vi "Autonomous Independent.vi"() -> ()   [LabVIEW 2015]
doc: "This VI is called when autonomous begins, and will automatically be terminated when autonomous ends. You can carry out timed or sensor driven robot movement independently without needing to return to the caller."
uses:
  <vilib>/Rock Robotics/SystemInterfaces/i2clib/i2c_bus.ctl
  <vilib>/Rock Robotics/Network Tables/NT Read String.vi
  <vilib>/Rock Robotics/WPI/Utilities/WPI_GetSetVariantRefNum.vi
  navX-MXP-LabVIEW/navX Library v2/navX Library v2.lvlib
panel:
  in  "array":bool[](array[boolean])
  in  "Distance (ft) 2":dbl
  in  "Angle (degrees)":dbl format="%.2f"
  in  "Distance (ft)":dbl
  # "Go this far"
  # "Turn thusly"
  # "Be sure to right-click and choose Data Operations>>Make Current Value default if you want to save the array values with the VI"
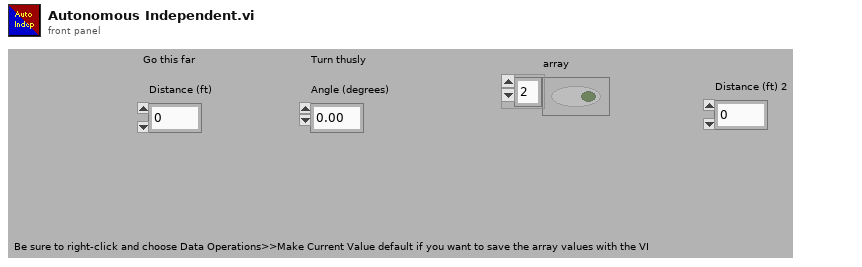
[diagram p1: front panel]
types:
  T1 = typedef "i2c_bus.ctl" = enum16{"I2C On-Board", "I2C MXP", "Invalid"}
  T2 = typedef "navX Library v2.lvlib/Z900_navX_DeviceTypeDef.ctl" = cluster{"Interface":cluster{"Protocol":T3, "Update Rate (4Hz-60Hz)":u8, "navX Open TypeDef":variant}, "Notify Packet":refnum<notifier>, "Loop VI Refnum":refnum<vi>, "Ready to Close Occurrence Refnum":refnum<k4>}
  T3 = typedef "navX Library v2.lvlib/Z900_navX_ProtocolTypeDef.ctl" = enum16{"SERIAL", "I2C", "SPI"}
  T4 = typedef "WPI_RobotDriveDevRef.ctl" = cluster{"DevStatus":errorcluster, "Motors[]":T5[], "Square Inputs":bool, "Max Output":dbl}
  T5 = typedef "WPI_MotorControlDeviceRef.ctl" = cluster{"DeviceStatus":errorcluster, "Type":T6, "PWM":cluster{"PWM Channel":T7, "DeadBand":T8}, "CAN":cluster{"Device Number":u8, "Control Mode":T9, "Semaphore":T10, "Max Vout":dbl, "TalonSRX Control Mode":T11}, "Invert":bool}
  T6 = typedef "WPI_MotorControlType.ctl" = enum16{"PWM", "CAN", "CANTalonSRX"}
  T7 = typedef "FPGA_DIOPWMChannel.ctl" = enum8{"PWM 0", "PWM 1", "PWM 2", "PWM 3", "PWM 4", "PWM 5", "PWM 6", "PWM 7", "PWM 8", "PWM 9", "PWM MXP 0", "PWM MXP 1", "PWM MXP 2", "PWM MXP 3", "PWM MXP 4", "PWM MXP 5", "PWM MXP 6", "PWM MXP 7", "PWM MXP 8", "PWM MXP 9", "Invalid"}
  T8 = typedef "WPI_PWMDeadband.ctl" = cluster{"Name":string, "maxPositivePwm":i32, "minPositivePwm":i32, "centerPwm":i32, "maxNegativePwm":i32, "minNegativePwm":i32, "angularRange":u16}
  T9 = typedef "WPI_CANJaguar_ControlMode.ctl" = enum8{"Percent VBus", "Current", "Speed", "Position", "Voltage"}
  T10 = typedef "Semaphore RefNum" = refnum<k1>
  T11 = typedef "WPI_CANTalonSRX_APIControlMode.ctl" = enum8{"Percent VBus", "Speed", "Position", "Slave", "Unchanged / Invalid", "Voltage Compensation", "Current", "Motion Profile"}
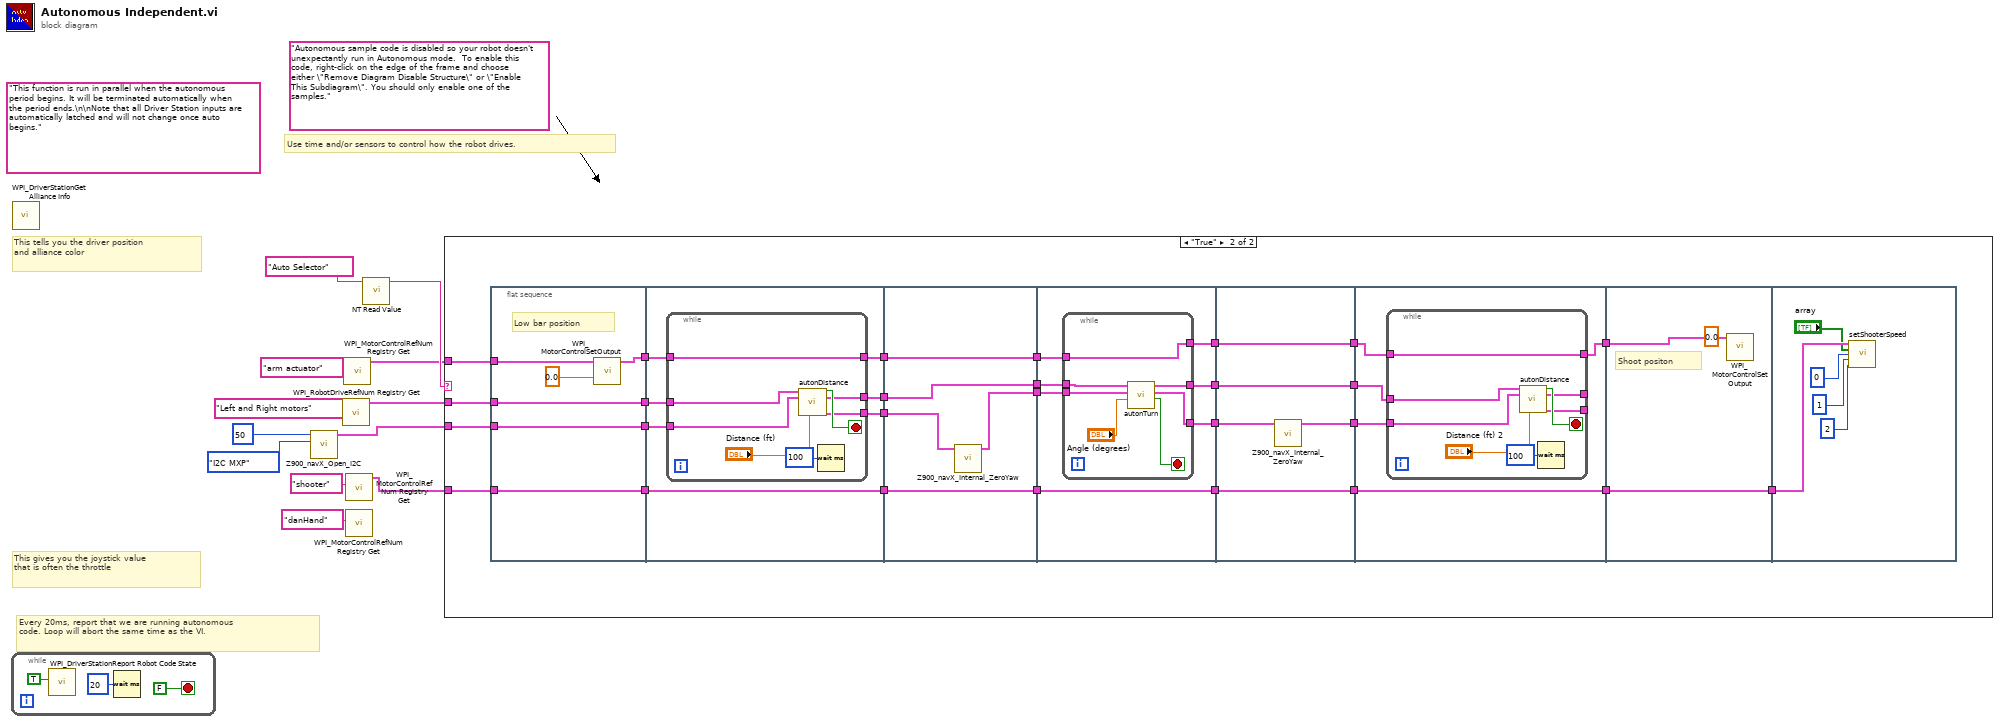
[diagram p0: block diagram]
diagram:
  (unwired) "Autonomous sample code is disabled so your robot doesn't unexpectantly run in Autonomous mode.  To enable this code, right-click on the edge of the frame and choose either \"Remove Diagram Disable Structure\" or \"Enable This Subdiagram\". You should only enable one of the samples."
  (unwired) "This function is run in parallel when the autonomous period begins. It will be terminated automatically when the period ends.\n\nNote that all Driver Station inputs are automatically latched and will not change once auto begins."
  # "Every 20ms, report that we are running autonomous\ncode. Loop will abort the same time as the VI."
  # "This gives you the joystick value\nthat is often the throttle"
  # "Use time and/or sensors to control how the robot drives."
  # "This tells you the driver position\nand alliance color"
  n1 = while {
    stop <- FALSE stop-if-true
    n2 = call <vilib>:"WPI_DriverStationReport Robot Code State.vi"("Autonomous"=TRUE) -> ()  [unwired: 10 in, 1 out]
    n3 = Wait (ms)(milliseconds to wait=u32 20) -> ()  [unwired: 1 out]
  }
  n4 = call <vilib>:"WPI_DriverStationGet Alliance Info.vi"() -> ()  [unwired: 12 out]
  n5 = call "Z900_navX_Open_I2C.vi"("I2C Bus"=i2c_bus."I2C MXP", "Update Rate (4Hz-60Hz)"=u8 50) -> ("navX Device"=w3:T2)  [unwired: 8 in, 1 out]
  n6 = call <vilib>:"WPI_RobotDriveRefNum Registry Get.vi"("refnum name"="Left and Right motors") -> ("RobotDriveDevRef"=w9:T4)  [unwired: 9 in, 1 out]
  n7 = call <vilib>:"WPI_MotorControlRefNum Registry Get.vi"("refnum name"="arm actuator") -> ("MotorControlDevRef"=w7:T5)  [unwired: 9 in, 1 out]
  n8 = call <vilib>:"WPI_MotorControlRefNum Registry Get.vi"("refnum name"="shooter") -> ("MotorControlDevRef"=w4:T5)  [unwired: 9 in, 1 out]
  n9 = call <vilib>:"WPI_MotorControlRefNum Registry Get.vi"("refnum name"="danHand") -> ()  [unwired: 9 in, 2 out]
  n10 = call-poly <vilib>:"NT Read Value.vi"("Name"="Auto Selector") -> ("String"=w11:string)  [unwired: 9 in, 1 out]
  n11 = case shown="\"True\"" w11 {
    tunnel: w9 -> [_ w42]
    tunnel: w3 -> [_ w41]
    tunnel: w7 -> [_ w24]
    tunnel: w4 -> [_ w23]
    frame "False", Default {
    }
    frame "True" {
      n12 = flat-sequence {
        tunnel: w41 -> [w47]
        tunnel: w42 -> [w48]
        tunnel: [w48] -> w27
        tunnel: [w47] -> w26
        tunnel: [w46] -> w25
        tunnel: w24 -> [w45]
        tunnel: w23 -> [w44]
        tunnel: [w44] -> w22
        tunnel: [w53] -> w40
        tunnel: [w52] -> w37
        tunnel: [w51] -> w35
        tunnel: w27 -> [w55]
        tunnel: w26 -> [w54]
        tunnel: w25 -> [w50]
        tunnel: w22 -> [w49]
        tunnel: [w49] -> w21
        tunnel: w40 -> [w65]
        tunnel: [w64] -> w39
        tunnel: [w68] -> w38
        tunnel: w37 -> [w68]
        tunnel: [w67] -> w36
        tunnel: w35 -> [w67]
        tunnel: w21 -> [w66]
        tunnel: [w66] -> w20
        tunnel: w39 -> [w75]
        tunnel: w38 -> [w74]
        tunnel: [w73] -> w33
        tunnel: w36 -> [w72]
        tunnel: [w71] -> w31
        tunnel: [w70] -> w29
        tunnel: w20 -> [w69]
        tunnel: [w69] -> w19
        tunnel: w33 -> [w87]
        tunnel: [w87] -> w32
        tunnel: w31 -> [w86]
        tunnel: [w86] -> w30
        tunnel: w29 -> [w84]
        tunnel: [w83] -> w28
        tunnel: w19 -> [w85]
        tunnel: [w85] -> w18
        tunnel: w32 -> [w92]
        tunnel: [w89] -> w34
        tunnel: w30 -> [w91]
        tunnel: w28 -> [w90]
        tunnel: w18 -> [w88]
        tunnel: [w88] -> w17
        tunnel: w34 -> [w103]
        tunnel: w17 -> [w102]
        tunnel: [w102] -> w16
        tunnel: w16 -> [w108]
        frame #0 {
          # "Low bar position"
          n13 = call <vilib>:"WPI_MotorControlSetOutput.vi"("Output"=0.0, "MotorControlDevRef"=w45) -> ("MotorControlDevRef"=w46:T5)  [unwired: 7 in, 2 out]
        }
        frame #1 {
          n14 = while {
            tunnel: w55 -> [w60]
            tunnel: w54 -> [w59]
            tunnel: [w58] -> w53
            tunnel: [w57] -> w52
            tunnel: [w56] -> w51
            tunnel: w50 -> [w56]
            stop <- w63 stop-if-true
            n15 = call "autonDistance.vi"("RobotDriveDevRef"=w60, "navX Device"=w59, "Numeric"="Distance (ft)") -> ("s? t:f"=w63:bool, "RobotDriveDevRef 2"=w57:T4, "navX Device 2"=w58:T2)  [unwired: 8 in, 2 out]
            n16 = Wait (ms)(milliseconds to wait=u32 100) -> ()  [unwired: 1 out]
          }
        }
        frame #2 {
          n17 = call "Z900_navX_Internal_ZeroYaw.vi"("navX Device"=w65) -> ("navX Device"=w64:T2)  [unwired: 7 in, 3 out]
        }
        frame #3 {
          n18 = while {
            tunnel: w75 -> [w82]
            tunnel: w74 -> [w81]
            tunnel: [w78] -> w73
            tunnel: w72 -> [w78]
            tunnel: [w77] -> w71
            tunnel: [w76] -> w70
            stop <- w79 stop-if-true
            n19 = call "autonTurn.vi"("setpoint"="Angle (degrees)", "navX Device"=w82, "RobotDriveDevRef 2"=w81) -> ("end"=w79:bool, "navX Device 2"=w76:T2, "RobotDriveDevRef"=w77:T4)  [unwired: 6 in]
          }
        }
        frame #4 {
          n20 = call "Z900_navX_Internal_ZeroYaw.vi"("navX Device"=w84) -> ("navX Device"=w83:T2)  [unwired: 7 in, 3 out]
        }
        frame #5 {
          n21 = while {
            tunnel: w91 -> [w97]
            tunnel: w90 -> [w96]
            tunnel: [w95] -> _
            tunnel: [w94] -> _
            tunnel: [w93] -> w89
            tunnel: w92 -> [w93]
            stop <- w100 stop-if-true
            n22 = call "autonDistance.vi"("RobotDriveDevRef"=w97, "navX Device"=w96, "Numeric"="Distance (ft) 2") -> ("s? t:f"=w100:bool, "RobotDriveDevRef 2"=w94:T4, "navX Device 2"=w95:T2)  [unwired: 8 in, 2 out]
            n23 = Wait (ms)(milliseconds to wait=u32 100) -> ()  [unwired: 1 out]
          }
        }
        frame #6 {
          # "Shoot positon"
          n24 = call <vilib>:"WPI_MotorControlSetOutput.vi"("Output"=0.0, "MotorControlDevRef"=w103) -> ()  [unwired: 7 in, 3 out]
        }
        frame #7 {
          n25 = call "setShooterSpeed.vi"("CAN Talon SRX Ref"=w108, "array"="array", "Intake Button"=0, "Shoot Button"=1, "Reverse Button"=2) -> ()  [unwired: 11 in]
        }
      }
    }
  }
